vi "control systems for stability analysis.vi"() -> ()   [LabVIEW 2013]
uses:
  <vilib>/addons/Control Design/_Model Construction/Data Typedefs.llb/CD frequency specs.ctl
  <vilib>/addons/Control Design/_Model Construction/Data Typedefs.llb/CD Margin Data.ctl
  <vilib>/addons/Control Design/_Model Construction/Model Creation.llb/Model Creation SubVI/cd_Create Transfer Function Model.vi
  <vilib>/addons/Control Design/_Model Conversions/Model Type.llb/Model Conversion SubVI/cd_Convert Transfer Function to State-Space Model.vi
  <vilib>/addons/Control Design/_Dynamic Analysis/Dynamic Analysis.llb/Dynamic Analysis subVI/cd_Stability (State-Space).vi
  <vilib>/addons/Control Design/_Dynamic Analysis/Dynamic Analysis.llb/Dynamic Analysis subVI/cd_DC Gain (State-Space).vi
  <vilib>/addons/Control Design/_Dynamic Analysis/Dynamic Analysis.llb/Dynamic Analysis subVI/cd_Damping Ratio and Natural Frequency (State-Space).vi
  <vilib>/addons/Control Design/_Model Delay/Model Delay.llb/Model Delay subVIs/cd_Distribute Delays (SS).vi
  <vilib>/addons/Control Design/_Model Delay/Model Delay.llb/Model Delay subVIs/cd_Total Delay (State Space).vi
  <vilib>/addons/Control Design/_Dynamic Analysis/Dynamic Analysis.llb/Dynamic Analysis subVI/cd_Transmission Zeros (State-Space).vi
  <vilib>/addons/Control Design/_Dynamic Analysis/Dynamic Analysis.llb/Dynamic Analysis subVI/cd_Poles (State-Space).vi
  <vilib>/addons/Control Design/_Dynamic Analysis/Dynamic Analysis.llb/Dynamic Analysis subVI/cd_Pole-Zero Map (State-Space).vi
  <vilib>/addons/Control Design/_Frequency Response Analysis/Frequency Response.llb/Frequency Response subVI/cd_Bode (State Space).vi
  <vilib>/addons/Control Design/_Frequency Response Analysis/Frequency Response.llb/Frequency Response subVI/cd_Nyquist (State-Space).vi
  <vilib>/addons/Control Design/_Time Response Analysis/Time Response.llb/Time Response subVI/cd_Step Response (State-Space).vi
  <vilib>/addons/Control Design/_Dynamic Analysis/Dynamic Analysis.llb/Dynamic Analysis subVI/cd_Root Locus (State-Space).vi
  <vilib>/addons/Control Design/_Utility/Model Viewer.llb/Model Viewer SubVI/cd_Draw State-Space Equation (SS).vi
  <vilib>/addons/Control Design/_Utility/Model Viewer.llb/Model Viewer SubVI/cd_Draw Transfer Function Equation (TF).vi
  <vilib>/addons/Control Design/_Frequency Response Analysis/Frequency Response.llb/Frequency Response subVI/cd_Bandwidth (State-Space).vi
  <vilib>/addons/Control Design/_Frequency Response Analysis/Frequency Response.llb/Frequency Response subVI/cd_Gain and Phase Margin (State-Space).vi
  <vilib>/addons/Control Design/_Model Construction/NI_LinSys_Model Creation.lvlib
  <vilib>/addons/Control Design/_Utility/NI_CD_Model Viewer.lvlib
  <vilib>/addons/Control Design/_Model Conversions/NI_CD_Model Type.lvlib
  <vilib>/addons/Control Design/_Dynamic Analysis/NI_CD_Dynamic Analysis.lvlib
  <vilib>/addons/Control Design/_Time Response Analysis/NI_CD_Time Response.lvlib
  <vilib>/addons/Control Design/_Frequency Response Analysis/NI_CD_Frequency Response.lvlib
  <vilib>/addons/Control Design/_State-Space Analysis/NI_CD_State-Space Analysis.lvlib
  <vilib>/addons/Control Design/_Model Delay/NI_CD_Model Delay.lvlib
  <vilib>/addons/Control Design/_Model Construction/NI_LinSys_Data Typedefs.lvlib
panel:
  out "Transport Delays":dbl[][](array[numeric]) format="%.2f"
  out "Output Delays":dbl[](array[numeric]) format="%.2f"
  in  "Magnitude Scale":enum16{"linear", "dB"}(ring)=enum."dB"
  out "Gain and Phase Margins":T1 {"Phase Margin" format="%#.4g"; "P.M. Frequency" format="%#.4g"; "Gain Margin" format="%#.4g"; "G.M. Frequency" format="%#.4g"}
  out "phase plot":cluster{"W":dbl[], "Magnitude":dbl[]}[](graph)
  out "Magnitude plot":cluster{"W":dbl[], "Magnitude":dbl[]}[](graph)
  in  "Magnitude Drop (dB)":dbl=-3.0 format="%.2f"
  out "Bandwidth":dbl=nan format="%.4f"
  in  "Frequency Unit":enum16{"Hz", "rad/s"}(ring)=enum."rad/s"
  in  "Frequency Range":T2={"Initial frequency"=-1.0, "Final frequency"=-1.0, "Minimum number of points"=-1, "Frequency Unit"=enum."rad/s"} {"Final frequency" format="%.2f"; "Initial frequency" format="%.2f"}
  out "Natural Frequencies":dbl[](array[numeric]) format="%.2f"
  out "Stability of the system":T3(ring)=enum."undetermined"
  out "DC Gain":dbl[][](array[numeric]) format="%#.8g"
  out "Damping Ratios":dbl[](array[numeric]) format="%.2f"
  out "Input Delays":dbl[](array[numeric]) format="%.2f"
  out "Total Delay":dbl[][](array[numeric]) format="%.4f"
  out "Observability  Matrix":dbl[][](array[numeric]) format="%#.2g"
  out "Controllability Matrix":dbl[][](array[numeric])=[[1.0, 0.0, 6.0], [0.0, 1.0, -1.0], [0.0, 0.0, 0.0]] format="%.2f"
  out "Zeros":cdb[](array[numeric]) format="%.4e"
  out "Poles":cdb[](array[numeric]) format="%.3f"
  out "pole zero map":cluster{dbl[], dbl[]}[](graph)
  out "Bode Magnitude":cluster{"W":dbl[], "Magnitude":dbl[]}[](graph)
  out "Nyquist Plot":cluster{"W":dbl[], "Magnitude":dbl[]}[](graph)
  out "Step Response Graph":cluster{"time":dbl[], dbl[]}[](graph)
  out "Root Locus Graph":cluster{dbl[], dbl[]}[](graph)
  out "State space  matrix":picture
  in  "Denominator part":dbl[](array[numeric])
  in  "Numerator part":dbl[](array[numeric])
  out "Transfer Function in S Domain":picture
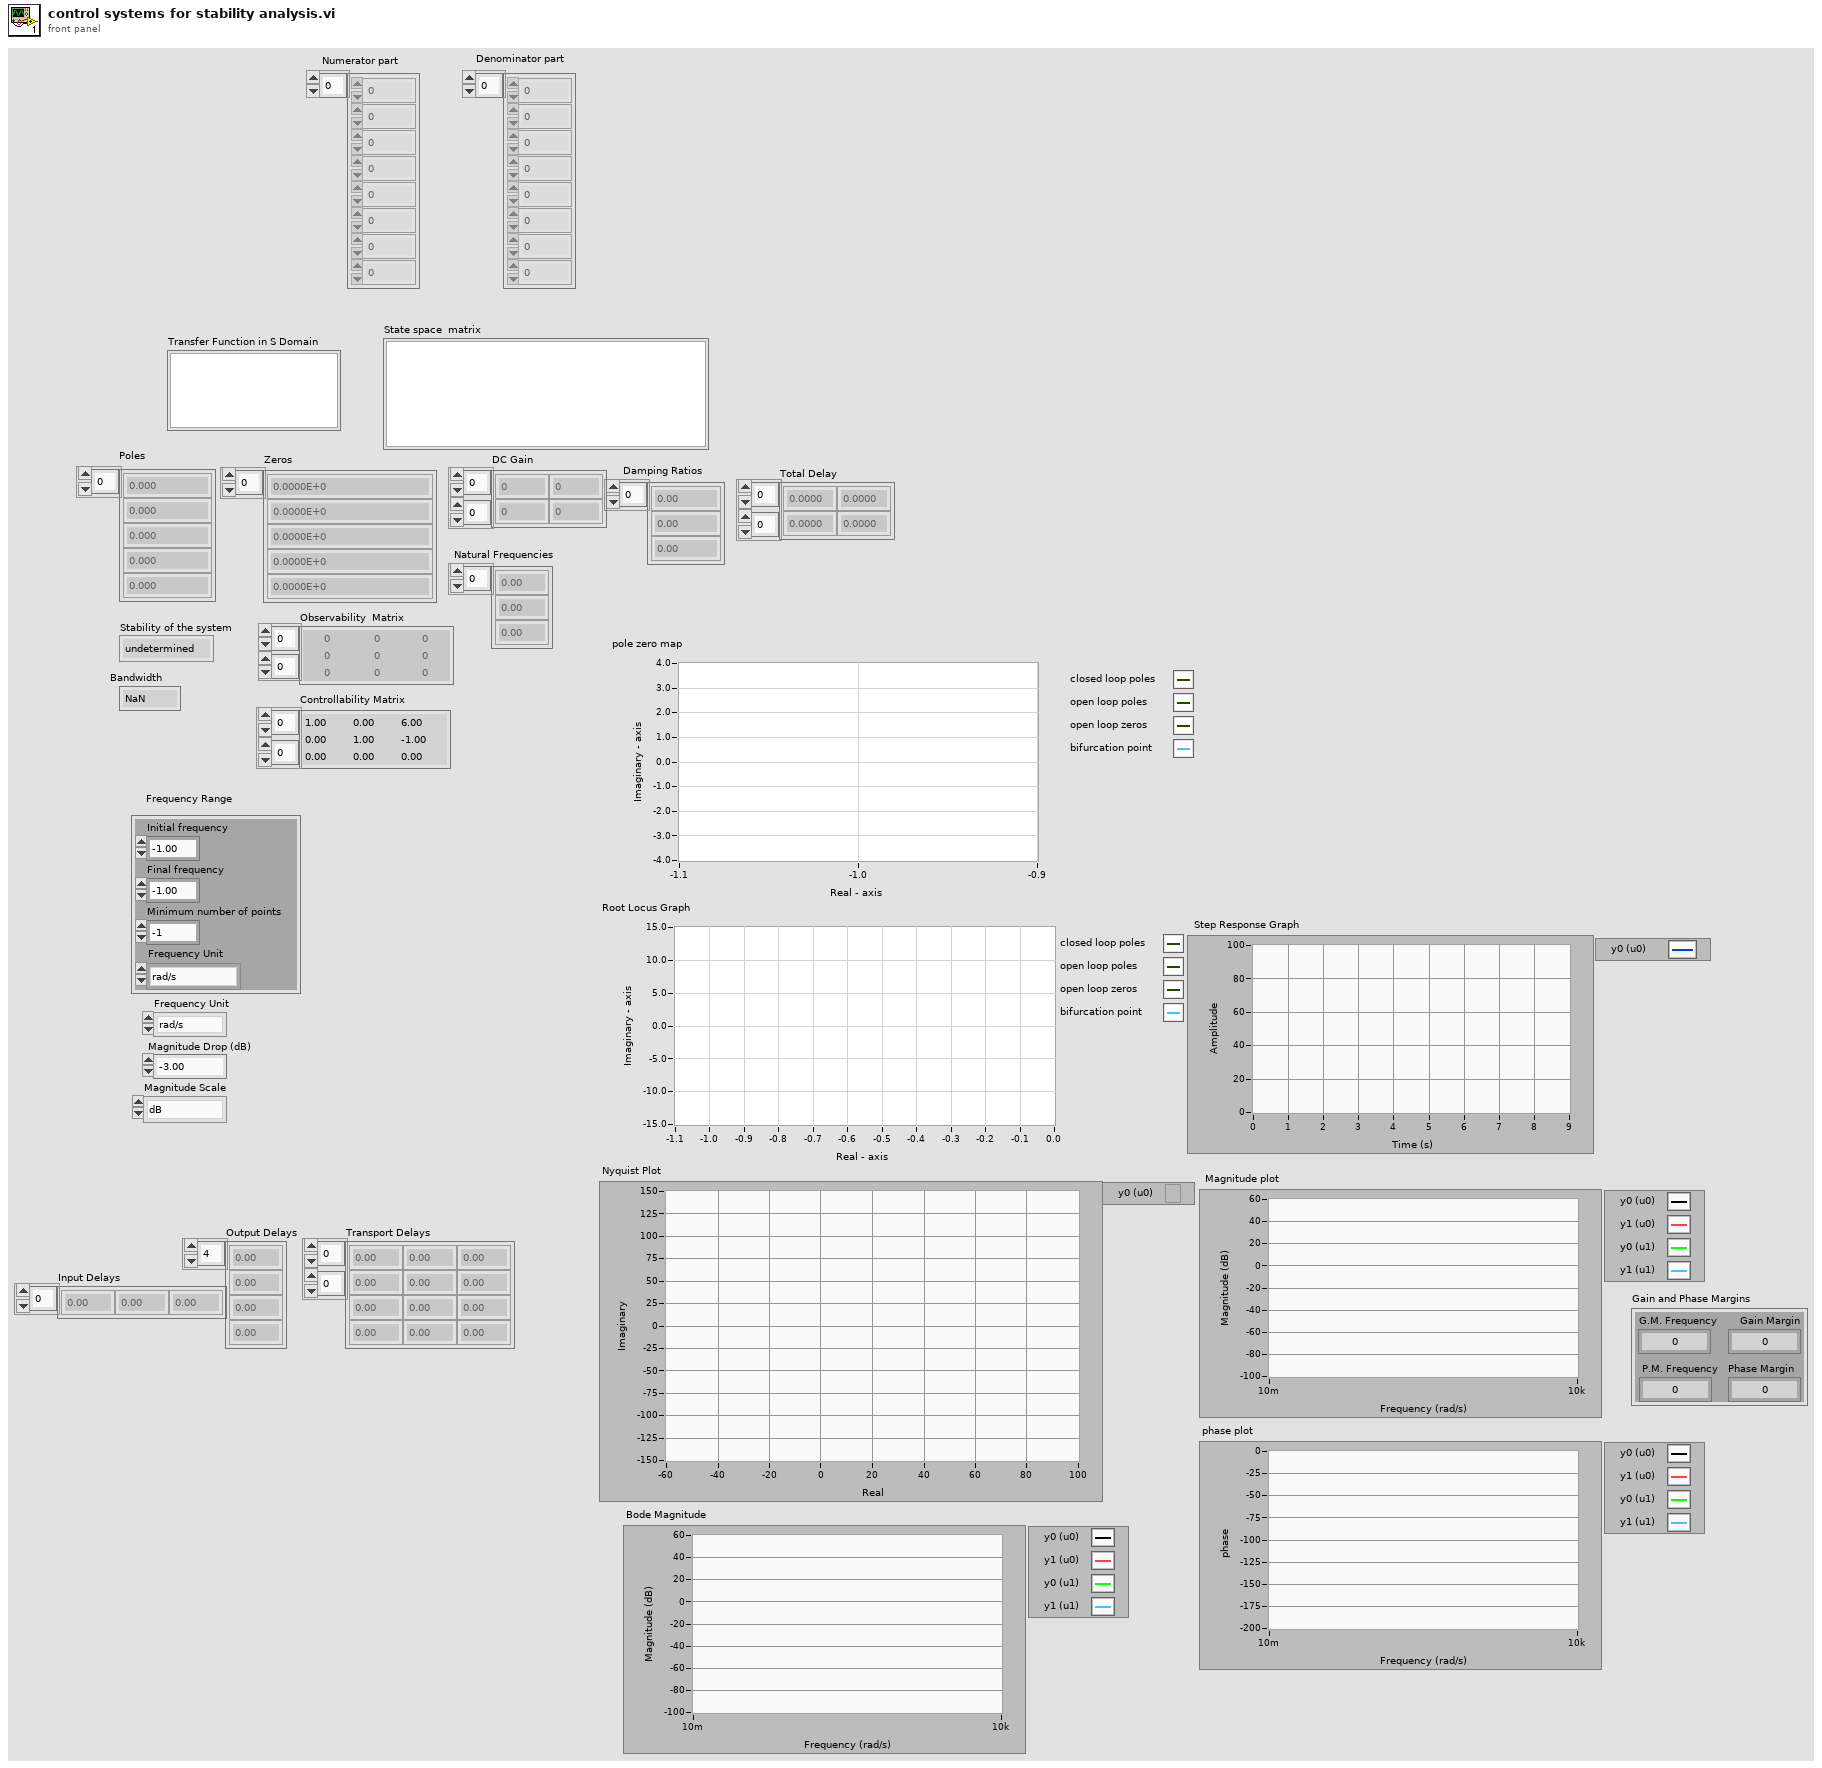
[diagram p1: front panel]
types:
  T1 = typedef "NI_LinSys_Data Typedefs.lvlib/CD Margin Data.ctl" = cluster{"G.M. Frequency":dbl, "Gain Margin":dbl, "P.M. Frequency":dbl, "Phase Margin":dbl}
  T2 = typedef "NI_LinSys_Data Typedefs.lvlib/CD frequency specs.ctl" = cluster{"Initial frequency":dbl, "Final frequency":dbl, "Minimum number of points":i32, "Frequency Unit":enum16{"Hz", "rad/s"}}
  T3 = enum16{"stable", "marginally stable", "unstable", "undetermined"}
  T4 = typedef "NI_LinSys_Model Typedefs.lvlib/CD Transfer Function Model (MIMO).ctl" = cluster{"properties":T5, "transfer function(s)":T6[][]}
  T5 = typedef "NI_LinSys_Model Typedefs.lvlib/CD General Elements.ctl" = cluster{"Model name":string, "Input names":string[], "Output names":string[], "Input Delays":dbl[], "Output Delays":dbl[], "Sampling Time":dbl, "Notes":string}
  T6 = typedef "NI_LinSys_Model Typedefs.lvlib/CD Transfer Function Model (SISO).ctl" = cluster{"Numerator":dbl[], "Denominator":dbl[], "delay":dbl}
  T7 = typedef "NI_LinSys_Model Typedefs.lvlib/CD State Space Model (MIMO).ctl" = cluster{"properties":T5, "A":dbl[][], "B":dbl[][], "C":dbl[][], "D":dbl[][], "StateNames":string[], "Transport Delay":dbl[][]}
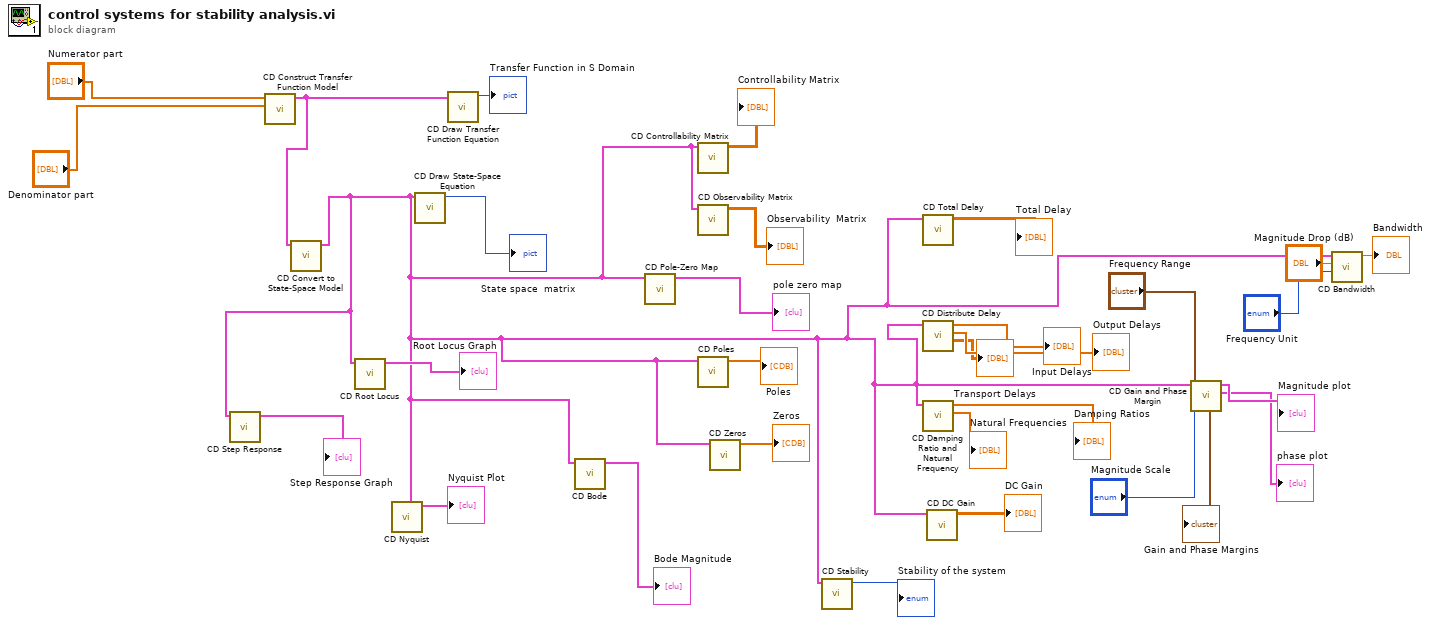
[diagram p0: block diagram]
diagram:
  n1 = call-poly <vilib>:"CD Construct Transfer Function Model.vi"("Denominator"="Denominator part", "Numerator"="Numerator part") -> ("Transfer Function Model"=w11:T4)  [unwired: 8 in, 1 out]
  n2 = call-poly <vilib>:"CD Convert to State-Space Model.vi"("Transfer Function Model"=w11) -> ("State-Space Model"=w3:T7)  [unwired: 9 in, 1 out]
  n3 = call-poly <vilib>:"CD Step Response.vi"("State-Space Model"=w3) -> ("Step Response Graph"=→"Step Response Graph":cluster{"time":dbl[], dbl[]}[])  [unwired: 7 in, 3 out]
  n4 = call-poly <vilib>:"CD Root Locus.vi"("State-Space Model"=w3) -> ("Root Locus Graph"=→"Root Locus Graph":cluster{dbl[], dbl[]}[])  [unwired: 7 in, 3 out]
  n5 = call-poly <vilib>:"CD Nyquist.vi"("State-Space Model"=w3) -> ("Nyquist Plot"=→"Nyquist Plot":cluster{"W":dbl[], "Magnitude":dbl[]}[])  [unwired: 8 in, 2 out]
  n6 = call-poly <vilib>:"CD Draw State-Space Equation.vi"("State-Space Model"=w3) -> ("Equation"=→"State space  matrix":picture)  [unwired: 8 in, 2 out]
  n7 = call-poly <vilib>:"CD Draw Transfer Function Equation.vi"("Transfer Function Model"=w11) -> ("Equation"=→"Transfer Function in S Domain":picture)  [unwired: 8 in, 2 out]
  n8 = call-poly <vilib>:"CD Bode.vi"("State-Space Model"=w3) -> ("Bode Magnitude"=→"Bode Magnitude":cluster{"W":dbl[], "Magnitude":dbl[]}[])  [unwired: 6 in, 4 out]
  n9 = call-poly <vilib>:"CD Pole-Zero Map.vi"("State-Space Model"=w3) -> ("Pole-Zero Map"=→"pole zero map":cluster{dbl[], dbl[]}[])  [unwired: 7 in, 3 out]
  n10 = call <vilib>:"CD Controllability Matrix.vi"("State-Space Model"=w3) -> ("Controllability Matrix"=→"Controllability Matrix":dbl[][])  [unwired: 7 in, 3 out]
  n11 = call <vilib>:"CD Observability Matrix.vi"("State-Space Model"=w3) -> ("Observability  Matrix"=→"Observability  Matrix":dbl[][])  [unwired: 7 in, 3 out]
  n12 = call-poly <vilib>:"CD Poles.vi"("State-Space Model"=w3) -> ("Poles"=→"Poles":cdb[])  [unwired: 9 in, 1 out]
  n13 = call-poly <vilib>:"CD Zeros.vi"("State-Space Model"=w3) -> ("Zeros"=→"Zeros":cdb[])  [unwired: 9 in, 1 out]
  n14 = call-poly <vilib>:"CD Stability.vi"("State-Space Model"=w3) -> ("Stability"=→"Stability of the system":T3)  [unwired: 8 in, 2 out]
  n15 = call-poly <vilib>:"CD Total Delay.vi"("State-Space Model"=w3) -> ("Total Delay"=→"Total Delay":dbl[][])  [unwired: 9 in, 1 out]
  n16 = call-poly <vilib>:"CD Distribute Delay.vi"("State-Space Model"=w3) -> ("Transport Delays"=→"Transport Delays":dbl[][], "Output Delays"=→"Output Delays":dbl[], "Input Delays"=→"Input Delays":dbl[])  [unwired: 7 in, 1 out]
  n17 = call-poly <vilib>:"CD Damping Ratio and Natural Frequency.vi"("State-Space Model"=w3) -> ("Natural Frequencies"=→"Natural Frequencies":dbl[], "Damping Ratios"=→"Damping Ratios":dbl[])  [unwired: 7 in, 2 out]
  n18 = call-poly <vilib>:"CD DC Gain.vi"("State-Space Model"=w3) -> ("DC Gain"=→"DC Gain":dbl[][])  [unwired: 8 in, 2 out]
  n19 = call-poly <vilib>:"CD Gain and Phase Margin.vi"("Magnitude Scale"="Magnitude Scale", "Frequency Range"="Frequency Range", "State-Space Model"=w3) -> ("Gain and Phase Margins"=→"Gain and Phase Margins":T1, "Phase Plot"=→"phase plot":cluster{"W":dbl[], "Phase":dbl[]}[], "Magnitude Plot"=→"Magnitude plot":cluster{"W":dbl[], "Magnitude":dbl[]}[])  [unwired: 4 in, 2 out]
  n20 = call-poly <vilib>:"CD Bandwidth.vi"("Frequency Unit"="Frequency Unit", "Magnitude Drop (dB)"="Magnitude Drop (dB)", "State-Space Model"=w3) -> ("Bandwidth"=→"Bandwidth":dbl)  [unwired: 7 in, 1 out]
